vi "Register gRPC Messages.vi"(8 "error in (no error)":errorcluster, 11 "gRPC ID":T1) -> (0 "error out":errorcluster, 3 "gRPC ID Out":T1)   [LabVIEW 2021, in "NI_DAQmx_client.lvlib"]
uses:
  NI_DAQmx_client.lvlib
  <vilib>/gRPC/LabVIEW gRPC Library/Shared/grpcId.ctl
  <vilib>/gRPC/LabVIEW gRPC Library/Server API/typeDefs/Message Metadata.ctl
  <vilib>/gRPC/LabVIEW gRPC Library/Server API/typeDefs/Message Element Metadata.ctl
  <vilib>/gRPC/LabVIEW gRPC Library/Server API/typeDefs/Message Element Type.ctl
  <vilib>/gRPC/LabVIEW gRPC Library/Server API/typeDefs/Enum Metadata.ctl
  <vilib>/gRPC/LabVIEW gRPC Library/grpc-lvsupport-release.lvlib
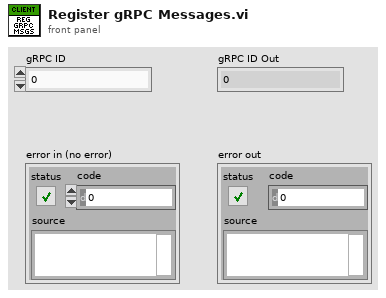
[diagram p1: front panel]
types:
  T1 = typedef "grpc-lvsupport-release.lvlib/grpcId.ctl" = u64
  T2 = typedef "grpc-lvsupport-release.lvlib/Enum Metadata.ctl" = cluster{"Version":i32, "Name":string, "Type Url":string, "Enum Values":string, "Allow Alias":bool}
  T3 = typedef "grpc-lvsupport-release.lvlib/Message Metadata.ctl" = cluster{"Version":i32, "Name":string, "Type Url":string, "Elements":T4[], "Has Oneof":bool}
  T4 = typedef "grpc-lvsupport-release.lvlib/Message Element Metadata.ctl" = cluster{"Field Name":string, "Embedded Message Name":string, "Protobuf Index":i32, "MessageElementType":T5, "Repeated":bool, "Is in Oneof":bool, "Oneof Container Name":string}
  T5 = typedef "grpc-lvsupport-release.lvlib/Message Element Type.ctl" = enum32{"Int32Value", "FloatValue", "DoubleValue", "BoolValue", "StringValue", "MessageValue", "Int64Value", "UInt32Value", "UInt64Value", "EnumValue", "Bytes", "Fixed64", "Fixed32", "SFixed64", "SFixed32", "SInt64", "SInt32"}
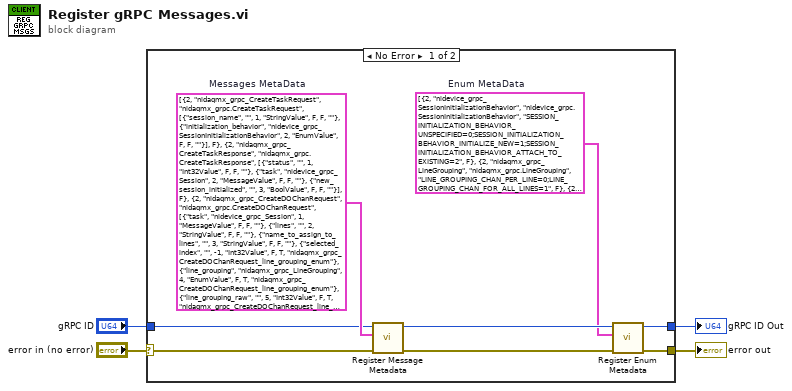
[diagram p0: block diagram]
diagram:
  n1 = case shown="No Error" "error in (no error)" {
    selector: "error in (no error)" -> [w10 w13]
    tunnel: [w9 w12] -> w1
    tunnel: [w6 w13] -> w4
    tunnel: "gRPC ID" -> [w9 w12]
    frame No Error {
      w5 = T2[] [{"Version"=2, "Name"="nidevice_grpc_SessionInitializationBehavior", "Type Url"="nidevice_grpc.SessionInitializationBehavior", "Enum Values"="SESSION_INITIALIZATION_BEHAVIOR_UNSPECIFIED=0;SESSION_INITIALIZATION_BEHAVIOR_INITIALIZE_NEW=1;SESSION_INITIALIZATION_BEHAVIOR_ATTACH_TO_EXISTING=2", "Allow Alias"=FALSE}, {"Version"=2, "Name"="nidaqmx_grpc_LineGrouping", "Type Url"="nidaqmx_grpc.LineGrouping", "Enum Values"="LINE_GROUPING_CHAN_PER_LINE=0;LINE_GROUPING_CHAN_FOR_ALL_LINES=1", "Allow Alias"=FALSE}, {"Version"=2, "Name"="nidaqmx_grpc_FrequencyUnits3", "Type Url"="nidaqmx_grpc.FrequencyUnits3", "Enum Values"="FREQUENCY_UNITS3_UNSPECIFIED=0;FREQUENCY_UNITS3_HZ=10373;FREQUENCY_UNITS3_TICKS=10304;FREQUENCY_UNITS3_FROM_CUSTOM_SCALE=10065", "Allow Alias"=FALSE}, {"Version"=2, "Name"="nidaqmx_grpc_Edge1", "Type Url"="nidaqmx_grpc.Edge1", "Enum Values"="EDGE1_UNSPECIFIED=0;EDGE1_RISING=10280;EDGE1_FALLING=10171", "Allow Alias"=FALSE}, {"Version"=2, "Name"="nidaqmx_grpc_CounterFrequencyMethod", "Type Url"="nidaqmx_grpc.CounterFrequencyMethod", "Enum Values"="COUNTER_FREQUENCY_METHOD_UNSPECIFIED=0;COUNTER_FREQUENCY_METHOD_LOW_FREQ_1_CTR=10105;COUNTER_FREQUENCY_METHOD_HIGH_FREQ_2_CTR=10157;COUNTER_FREQUENCY_METHOD_LARGE_RNG_2_CTR=10205;COUNTER_FREQUENCY_METHOD_DYN_AVG=16065", "Allow Alias"=FALSE}, {"Version"=2, "Name"="nidaqmx_grpc_GroupBy", "Type Url"="nidaqmx_grpc.GroupBy", "Enum Values"="GROUP_BY_GROUP_BY_CHANNEL=0;GROUP_BY_GROUP_BY_SCAN_NUMBER=1", "Allow Alias"=FALSE}, {"Version"=2, "Name"="nidaqmx_grpc_AcquisitionType", "Type Url"="nidaqmx_grpc.AcquisitionType", "Enum Values"="ACQUISITION_TYPE_UNSPECIFIED=0;ACQUISITION_TYPE_FINITE_SAMPS=10178;ACQUISITION_TYPE_CONT_SAMPS=10123;ACQUISITION_TYPE_HW_TIMED_SINGLE_POINT=12522", "Allow Alias"=FALSE}, {"Version"=2, "Name"="nidaqmx_grpc_TaskStringAttribute", "Type Url"="nidaqmx_grpc.TaskStringAttribute", "Enum Values"="TASK_STRING_ATTRIBUTE_UNSPECIFIED=0;TASK_ATTRIBUTE_CHANNELS=4723;TASK_ATTRIBUTE_NAME=4726;TASK_ATTRIBUTE_DEVICES=8974", "Allow Alias"=FALSE}, {"Version"=2, "Name"="nidaqmx_grpc_ChannelStringAttribute", "Type Url"="nidaqmx_grpc.ChannelStringAttribute", "Enum Values"="CHANNEL_STRING_ATTRIBUTE_UNSPECIFIED=0;CHANNEL_ATTRIBUTE_CI_CTR_TIMEBASE_SRC=323;CHANNEL_ATTRIBUTE_CO_CTR_TIMEBASE_SRC=825;CHANNEL_ATTRIBUTE_AI_THRMCPL_CJC_CHAN=4148;CHANNEL_ATTRIBUTE_CI_GPS_SYNC_SRC=4243;CHANNEL_ATTRIBUTE_AO_CUSTOM_SCALE_NAME=4488;CHANNEL_ATTRIBUTE_AI_CUSTOM_SCALE_NAME=6112;CHANNEL_ATTRIBUTE_CI_CUSTOM_SCALE_NAME=6302;CHANNEL_ATTRIBUTE_CI_FREQ_TERM=6306;CHANNEL_ATTRIBUTE_CI_PERIOD_TERM=6308;CHANNEL_ATTRIBUTE_CI_PULSE_WIDTH_TERM=6314;CHANNEL_ATTRIBUTE_CI_TWO_EDGE_SEP_FIRST_TERM=6317;CHANNEL_ATTRIBUTE_CI_TWO_EDGE_SEP_SECOND_TERM=6318;CHANNEL_ATTRIBUTE_CI_SEMI_PERIOD_TERM=6320;CHANNEL_ATTRIBUTE_CI_COUNT_EDGES_TERM=6343;CHANNEL_ATTRIBUTE_CO_PULSE_TERM=6369;CHANNEL_ATTRIBUTE_PHYSICAL_CHAN_NAME=6389;CHANNEL_ATTRIBUTE_CHAN_DESCR=6438;CHANNEL_ATTRIBUTE_AI_INPUT_SRC=8600;CHANNEL_ATTRIBUTE_CI_ENCODER_A_INPUT_TERM=8605;CHANNEL_ATTRIBUTE_CI_ENCODER_B_INPUT_TERM=8606;CHANNEL_ATTRIBUTE_CI_ENCODER_Z_INPUT_TERM=8607;CHANNEL_ATTRIBUTE_AI_TEDS_UNITS=8672;CHANNEL_ATTRIBUTE_CI_COUNT_EDGES_DIR_TERM=8673;CHANNEL_ATTRIBUTE_CI_FREQ_DIG_FLTR_TIMEBASE_SRC=8681;CHANNEL_ATTRIBUTE_CI_PERIOD_DIG_FLTR_TIMEBASE_SRC=8686;CHANNEL_ATTRIBUTE_CI_COUNT_EDGES_COUNT_DIR_DIG_FLTR_TIMEBASE_SRC=8691;CHANNEL_ATTRIBUTE_CI_COUNT_EDGES_DIG_FLTR_TIMEBASE_SRC=8696;CHANNEL_ATTRIBUTE_CI_ENCODER_A_INPUT_DIG_FLTR_TIMEBASE_SRC=8701;CHANNEL_ATTRIBUTE_CI_ENCODER_B_INPUT_DIG_FLTR_TIMEBASE_SRC=8706;CHANNEL_ATTRIBUTE_CI_ENCODER_Z_INPUT_DIG_FLTR_TIMEBASE_SRC=8711;CHANNEL_ATTRIBUTE_CI_PULSE_WIDTH_DIG_FLTR_TIMEBASE_SRC=8716;CHANNEL_ATTRIBUTE_CI_TWO_EDGE_SEP_FIRST_DIG_FLTR_TIMEBASE_SRC=8721;CHANNEL_ATTRIBUTE_CI_TWO_EDGE_SEP_SECOND_DIG_FLTR_TIMEBASE_SRC=8726;CHANNEL_ATTRIBUTE_CI_SEMI_PERIOD_DIG_FLTR_TIMEBASE_SRC=8731;CHANNEL_ATTRIBUTE_AO_DAC_REF_EXT_SRC=8786;CHANNEL_ATTRIBUTE_AO_DAC_OFFSET_EXT_SRC=8788;CHANNEL_ATTRIBUTE_CI_CTR_TIMEBASE_DIG_FLTR_TIMEBASE_SRC=8819;CHANNEL_ATTRIBUTE_CO_CTR_TIMEBASE_DIG_FLTR_TIMEBASE_SRC=8824;CHANNEL_ATTRIBUTE_AI_CHAN_CAL_OPERATOR_NAME=8867;CHANNEL_ATTRIBUTE_AI_CHAN_CAL_DESC=8868;CHANNEL_ATTRIBUTE_DI_DIG_FLTR_TIMEBASE_SRC=11988;CHANNEL_ATTRIBUTE_CI_PULSE_FREQ_TERM=12036;CHANNEL_ATTRIBUTE_CI_PULSE_FREQ_DIG_FLTR_TIMEBASE_SRC=12040;CHANNEL_ATTRIBUTE_CI_PULSE_TIME_TERM=12044;CHANNEL_ATTRIBUTE_CI_PULSE_TIME_DIG_FLTR_TIMEBASE_SRC=12048;CHANNEL_ATTRIBUTE_CI_PULSE_TICKS_TERM=12052;CHANNEL_ATTRIBUTE_CI_PULSE_TICKS_DIG_FLTR_TIMEBASE_SRC=12056;CHANNEL_ATTRIBUTE_CI_COUNT_EDGES_COUNT_RESET_TERM=12209;CHANNEL_ATTRIBUTE_CI_COUNT_EDGES_COUNT_RESET_DIG_FLTR_TIMEBASE_SRC=12213;CHANNEL_ATTRIBUTE_AI_ROSETTE_STRAIN_GAGE_STRAIN_CHANS=12283;CHANNEL_ATTRIBUTE_CI_TIMESTAMP_TERM=12345;CHANNEL_ATTRIBUTE_NAV_CUSTOM_SCALE_NAME=12348;CHANNEL_ATTRIBUTE_CI_DUTY_CYCLE_TERM=12429;CHANNEL_ATTRIBUTE_CI_DUTY_CYCLE_DIG_FLTR_TIMEBASE_SRC=12432;CHANNEL_ATTRIBUTE_CI_VELOCITY_ENCODER_A_INPUT_TERM=12509;CHANNEL_ATTRIBUTE_CI_VELOCITY_ENCODER_A_INPUT_DIG_FLTR_TIMEBASE_SRC=12514;CHANNEL_ATTRIBUTE_CI_VELOCITY_ENCODER_B_INPUT_TERM=12516;CHANNEL_ATTRIBUTE_CI_VELOCITY_ENCODER_B_INPUT_DIG_FLTR_TIMEBASE_SRC=12521;CHANNEL_ATTRIBUTE_CI_COUNT_EDGES_GATE_TERM=12526;CHANNEL_ATTRIBUTE_CI_COUNT_EDGES_GATE_DIG_FLTR_TIMEBASE_SRC=12531", "Allow Alias"=FALSE}, {"Version"=2, "Name"="nidaqmx_grpc_ChannelDoubleAttribute", "Type Url"="nidaqmx_grpc.ChannelDoubleAttribute", "Enum Values"="CHANNEL_DOUBLE_ATTRIBUTE_UNSPECIFIED=0;CHANNEL_ATTRIBUTE_AI_IMPEDANCE=98;CHANNEL_ATTRIBUTE_AI_AC_EXCIT_FREQ=257;CHANNEL_ATTRIBUTE_AO_GAIN=280;CHANNEL_ATTRIBUTE_AO_LOAD_IMPEDANCE=289;CHANNEL_ATTRIBUTE_CI_FREQ_MEAS_TIME=325;CHANNEL_ATTRIBUTE_CO_PULSE_FREQ_INITIAL_DELAY=665;CHANNEL_ATTRIBUTE_AI_ACCEL_SENSITIVITY=1682;CHANNEL_ATTRIBUTE_AI_FREQ_HYST=2068;CHANNEL_ATTRIBUTE_AI_FREQ_THRESH_VOLTAGE=2069;CHANNEL_ATTRIBUTE_CI_ANG_ENCODER_INITIAL_ANGLE=2177;CHANNEL_ATTRIBUTE_CI_ENCODER_Z_INDEX_VAL=2184;CHANNEL_ATTRIBUTE_AI_RVDT_SENSITIVITY=2307;CHANNEL_ATTRIBUTE_CI_LIN_ENCODER_DIST_PER_PULSE=2321;CHANNEL_ATTRIBUTE_CI_LIN_ENCODER_INITIAL_POS=2325;CHANNEL_ATTRIBUTE_AI_LVDT_SENSITIVITY=2361;CHANNEL_ATTRIBUTE_AI_STRAIN_GAGE_GAGE_FACTOR=2452;CHANNEL_ATTRIBUTE_AI_STRAIN_GAGE_POISSON_RATIO=2456;CHANNEL_ATTRIBUTE_AI_RTD_A=4112;CHANNEL_ATTRIBUTE_AI_RTD_B=4113;CHANNEL_ATTRIBUTE_AI_RTD_C=4115;CHANNEL_ATTRIBUTE_AI_RTD_R0=4144;CHANNEL_ATTRIBUTE_AI_THRMCPL_CJC_VAL=4150;CHANNEL_ATTRIBUTE_AI_THRMSTR_R1=4193;CHANNEL_ATTRIBUTE_CO_PULSE_DUTY_CYC=4470;CHANNEL_ATTRIBUTE_CO_PULSE_FREQ=4472;CHANNEL_ATTRIBUTE_AO_MAX=4486;CHANNEL_ATTRIBUTE_AO_MIN=4487;CHANNEL_ATTRIBUTE_AO_OUTPUT_IMPEDANCE=5264;CHANNEL_ATTRIBUTE_AI_MICROPHONE_SENSITIVITY=5430;CHANNEL_ATTRIBUTE_AI_RESOLUTION=5989;CHANNEL_ATTRIBUTE_AI_MAX=6109;CHANNEL_ATTRIBUTE_AI_MIN=6110;CHANNEL_ATTRIBUTE_AI_BRIDGE_NOM_RESISTANCE=6124;CHANNEL_ATTRIBUTE_AI_BRIDGE_INITIAL_VOLTAGE=6125;CHANNEL_ATTRIBUTE_AI_LEAD_WIRE_RESISTANCE=6126;CHANNEL_ATTRIBUTE_AI_CURRENT_SHUNT_RESISTANCE=6131;CHANNEL_ATTRIBUTE_AI_EXCIT_VAL=6133;CHANNEL_ATTRIBUTE_AI_ATTEN=6145;CHANNEL_ATTRIBUTE_AI_LOWPASS_CUTOFF_FREQ=6147;CHANNEL_ATTRIBUTE_AI_HIGHPASS_CUTOFF_FREQ=6151;CHANNEL_ATTRIBUTE_AI_BANDPASS_CENTER_FREQ=6156;CHANNEL_ATTRIBUTE_AI_BANDPASS_WIDTH=6158;CHANNEL_ATTRIBUTE_AI_NOTCH_CENTER_FREQ=6160;CHANNEL_ATTRIBUTE_AI_NOTCH_WIDTH=6162;CHANNEL_ATTRIBUTE_AI_RNG_HIGH=6165;CHANNEL_ATTRIBUTE_AI_RNG_LOW=6166;CHANNEL_ATTRIBUTE_AI_GAIN=6168;CHANNEL_ATTRIBUTE_AO_RESOLUTION=6188;CHANNEL_ATTRIBUTE_AO_DAC_RNG_LOW=6189;CHANNEL_ATTRIBUTE_AO_DAC_RNG_HIGH=6190;CHANNEL_ATTRIBUTE_AO_DAC_REF_VAL=6194;CHANNEL_ATTRIBUTE_AI_EXCIT_ACTUAL_VAL=6275;CHANNEL_ATTRIBUTE_AI_LOWPASS_SWITCH_CAP_EXT_CLK_FREQ=6277;CHANNEL_ATTRIBUTE_CI_MAX=6300;CHANNEL_ATTRIBUTE_CI_MIN=6301;CHANNEL_ATTRIBUTE_CI_CTR_TIMEBASE_RATE=6322;CHANNEL_ATTRIBUTE_CO_PULSE_HIGH_TIME=6330;CHANNEL_ATTRIBUTE_CO_PULSE_LOW_TIME=6331;CHANNEL_ATTRIBUTE_CO_PULSE_TIME_INITIAL_DELAY=6332;CHANNEL_ATTRIBUTE_CO_CTR_TIMEBASE_RATE=6338;CHANNEL_ATTRIBUTE_AI_THRMSTR_A=6345;CHANNEL_ATTRIBUTE_AI_THRMSTR_C=6346;CHANNEL_ATTRIBUTE_AI_THRMSTR_B=6347;CHANNEL_ATTRIBUTE_CI_PERIOD_MEAS_TIME=6445;CHANNEL_ATTRIBUTE_AI_BRIDGE_SHUNT_CAL_GAIN_ADJUST=6463;CHANNEL_ATTRIBUTE_DI_DIG_FLTR_MIN_PULSE_WIDTH=8663;CHANNEL_ATTRIBUTE_CI_FREQ_DIG_FLTR_MIN_PULSE_WIDTH=8680;CHANNEL_ATTRIBUTE_CI_FREQ_DIG_FLTR_TIMEBASE_RATE=8682;CHANNEL_ATTRIBUTE_CI_PERIOD_DIG_FLTR_MIN_PULSE_WIDTH=8685;CHANNEL_ATTRIBUTE_CI_PERIOD_DIG_FLTR_TIMEBASE_RATE=8687;CHANNEL_ATTRIBUTE_CI_COUNT_EDGES_COUNT_DIR_DIG_FLTR_MIN_PULSE_WIDTH=8690;CHANNEL_ATTRIBUTE_CI_COUNT_EDGES_COUNT_DIR_DIG_FLTR_TIMEBASE_RATE=8692;CHANNEL_ATTRIBUTE_CI_COUNT_EDGES_DIG_FLTR_MIN_PULSE_WIDTH=8695;CHANNEL_ATTRIBUTE_CI_COUNT_EDGES_DIG_FLTR_TIMEBASE_RATE=8697;CHANNEL_ATTRIBUTE_CI_ENCODER_A_INPUT_DIG_FLTR_MIN_PULSE_WIDTH=8700;CHANNEL_ATTRIBUTE_CI_ENCODER_A_INPUT_DIG_FLTR_TIMEBASE_RATE=8702;CHANNEL_ATTRIBUTE_CI_ENCODER_B_INPUT_DIG_FLTR_MIN_PULSE_WIDTH=8705;CHANNEL_ATTRIBUTE_CI_ENCODER_B_INPUT_DIG_FLTR_TIMEBASE_RATE=8707;CHANNEL_ATTRIBUTE_CI_ENCODER_Z_INPUT_DIG_FLTR_MIN_PULSE_WIDTH=8710;CHANNEL_ATTRIBUTE_CI_ENCODER_Z_INPUT_DIG_FLTR_TIMEBASE_RATE=8712;CHANNEL_ATTRIBUTE_CI_PULSE_WIDTH_DIG_FLTR_MIN_PULSE_WIDTH=8715;CHANNEL_ATTRIBUTE_CI_PULSE_WIDTH_DIG_FLTR_TIMEBASE_RATE=8717;CHANNEL_ATTRIBUTE_CI_TWO_EDGE_SEP_FIRST_DIG_FLTR_MIN_PULSE_WIDTH=8720;CHANNEL_ATTRIBUTE_CI_TWO_EDGE_SEP_FIRST_DIG_FLTR_TIMEBASE_RATE=8722;CHANNEL_ATTRIBUTE_CI_TWO_EDGE_SEP_SECOND_DIG_FLTR_MIN_PULSE_WIDTH=8725;CHANNEL_ATTRIBUTE_CI_TWO_EDGE_SEP_SECOND_DIG_FLTR_TIMEBASE_RATE=8727;CHANNEL_ATTRIBUTE_CI_SEMI_PERIOD_DIG_FLTR_MIN_PULSE_WIDTH=8730;CHANNEL_ATTRIBUTE_CI_SEMI_PERIOD_DIG_FLTR_TIMEBASE_RATE=8732;CHANNEL_ATTRIBUTE_AI_SOUND_PRESSURE_MAX_SOUND_PRESSURE_LVL=8762;CHANNEL_ATTRIBUTE_AO_DAC_OFFSET_VAL=8789;CHANNEL_ATTRIBUTE_CI_CTR_TIMEBASE_DIG_FLTR_MIN_PULSE_WIDTH=8818;CHANNEL_ATTRIBUTE_CI_CTR_TIMEBASE_DIG_FLTR_TIMEBASE_RATE=8820;CHANNEL_ATTRIBUTE_CO_CTR_TIMEBASE_DIG_FLTR_MIN_PULSE_WIDTH=8823;CHANNEL_ATTRIBUTE_CO_CTR_TIMEBASE_DIG_FLTR_TIMEBASE_RATE=8825;CHANNEL_ATTRIBUTE_AI_VOLTAGE_DB_REF=10672;CHANNEL_ATTRIBUTE_AI_SOUND_PRESSURE_DB_REF=10673;CHANNEL_ATTRIBUTE_AI_ACCEL_DB_REF=10674;CHANNEL_ATTRIBUTE_AO_FUNC_GEN_FREQ=10777;CHANNEL_ATTRIBUTE_AO_FUNC_GEN_AMPLITUDE=10778;CHANNEL_ATTRIBUTE_AO_FUNC_GEN_OFFSET=10779;CHANNEL_ATTRIBUTE_AO_FUNC_GEN_SQUARE_DUTY_CYCLE=10780;CHANNEL_ATTRIBUTE_AO_VOLTAGE_CURRENT_LIMIT=10781;CHANNEL_ATTRIBUTE_AO_FUNC_GEN_FM_DEVIATION=10787;CHANNEL_ATTRIBUTE_DO_OVERCURRENT_LIMIT=10885;CHANNEL_ATTRIBUTE_DO_OVERCURRENT_REENABLE_PERIOD=10887;CHANNEL_ATTRIBUTE_AI_PROBE_ATTEN=10888;CHANNEL_ATTRIBUTE_AI_DC_OFFSET=10889;CHANNEL_ATTRIBUTE_AI_EDDY_CURRENT_PROX_PROBE_SENSITIVITY=10942;CHANNEL_ATTRIBUTE_DI_DIG_FLTR_TIMEBASE_RATE=11989;CHANNEL_ATTRIBUTE_CI_PULSE_FREQ_DIG_FLTR_MIN_PULSE_WIDTH=12039;CHANNEL_ATTRIBUTE_CI_PULSE_FREQ_DIG_FLTR_TIMEBASE_RATE=12041;CHANNEL_ATTRIBUTE_CI_PULSE_TIME_DIG_FLTR_MIN_PULSE_WIDTH=12047;CHANNEL_ATTRIBUTE_CI_PULSE_TIME_DIG_FLTR_TIMEBASE_RATE=12049;CHANNEL_ATTRIBUTE_CI_PULSE_TICKS_DIG_FLTR_MIN_PULSE_WIDTH=12055;CHANNEL_ATTRIBUTE_CI_PULSE_TICKS_DIG_FLTR_TIMEBASE_RATE=12057;CHANNEL_ATTRIBUTE_AI_BRIDGE_SHUNT_CAL_SHUNT_CAL_A_RESISTANCE=12152;CHANNEL_ATTRIBUTE_AI_BRIDGE_SHUNT_CAL_SHUNT_CAL_A_ACTUAL_RESISTANCE=12153;CHANNEL_ATTRIBUTE_AI_BRIDGE_SHUNT_CAL_SHUNT_CAL_B_RESISTANCE=12154;CHANNEL_ATTRIBUTE_AI_BRIDGE_SHUNT_CAL_SHUNT_CAL_B_ACTUAL_RESISTANCE=12155;CHANNEL_ATTRIBUTE_AI_FORCE_IEPE_SENSOR_SENSITIVITY=12161;CHANNEL_ATTRIBUTE_AI_BRIDGE_INITIAL_RATIO=12166;CHANNEL_ATTRIBUTE_AI_BRIDGE_TWO_POINT_LIN_FIRST_ELECTRICAL_VAL=12170;CHANNEL_ATTRIBUTE_AI_BRIDGE_TWO_POINT_LIN_FIRST_PHYSICAL_VAL=12171;CHANNEL_ATTRIBUTE_AI_BRIDGE_TWO_POINT_LIN_SECOND_ELECTRICAL_VAL=12172;CHANNEL_ATTRIBUTE_AI_BRIDGE_TWO_POINT_LIN_SECOND_PHYSICAL_VAL=12173;CHANNEL_ATTRIBUTE_CI_COUNT_EDGES_COUNT_RESET_DIG_FLTR_MIN_PULSE_WIDTH=12212;CHANNEL_ATTRIBUTE_CI_COUNT_EDGES_COUNT_RESET_DIG_FLTR_TIMEBASE_RATE=12214;CHANNEL_ATTRIBUTE_AI_THRMCPL_LEAD_OFFSET_VOLTAGE=12216;CHANNEL_ATTRIBUTE_AI_FILTER_DELAY=12269;CHANNEL_ATTRIBUTE_AI_VELOCITY_IEPE_SENSOR_DB_REF=12277;CHANNEL_ATTRIBUTE_AI_VELOCITY_IEPE_SENSOR_SENSITIVITY=12278;CHANNEL_ATTRIBUTE_AI_ROSETTE_STRAIN_GAGE_ORIENTATION=12284;CHANNEL_ATTRIBUTE_AO_FILTER_DELAY_ADJUSTMENT=12402;CHANNEL_ATTRIBUTE_AI_FILTER_DELAY_ADJUSTMENT=12404;CHANNEL_ATTRIBUTE_AO_FILTER_DELAY=12405;CHANNEL_ATTRIBUTE_CI_DUTY_CYCLE_DIG_FLTR_MIN_PULSE_WIDTH=12431;CHANNEL_ATTRIBUTE_CI_DUTY_CYCLE_DIG_FLTR_TIMEBASE_RATE=12433;CHANNEL_ATTRIBUTE_CI_MAX_MEAS_PERIOD=12437;CHANNEL_ATTRIBUTE_CI_THRESH_VOLTAGE=12471;CHANNEL_ATTRIBUTE_AI_DIG_FLTR_LOWPASS_CUTOFF_FREQ=12481;CHANNEL_ATTRIBUTE_AI_DIG_FLTR_HIGHPASS_CUTOFF_FREQ=12482;CHANNEL_ATTRIBUTE_AI_DIG_FLTR_BANDPASS_CENTER_FREQ=12483;CHANNEL_ATTRIBUTE_AI_DIG_FLTR_BANDPASS_WIDTH=12484;CHANNEL_ATTRIBUTE_AI_DIG_FLTR_NOTCH_CENTER_FREQ=12485;CHANNEL_ATTRIBUTE_AI_DIG_FLTR_NOTCH_WIDTH=12486;CHANNEL_ATTRIBUTE_CI_VELOCITY_LIN_ENCODER_DIST_PER_PULSE=12507;CHANNEL_ATTRIBUTE_CI_VELOCITY_ENCODER_A_INPUT_DIG_FLTR_MIN_PULSE_WIDTH=12513;CHANNEL_ATTRIBUTE_CI_VELOCITY_ENCODER_A_INPUT_DIG_FLTR_TIMEBASE_RATE=12515;CHANNEL_ATTRIBUTE_CI_VELOCITY_ENCODER_B_INPUT_DIG_FLTR_MIN_PULSE_WIDTH=12520;CHANNEL_ATTRIBUTE_CI_VELOCITY_ENCODER_B_INPUT_DIG_FLTR_TIMEBASE_RATE=12522;CHANNEL_ATTRIBUTE_CI_VELOCITY_MEAS_TIME=12523;CHANNEL_ATTRIBUTE_CI_COUNT_EDGES_GATE_DIG_FLTR_MIN_PULSE_WIDTH=12530;CHANNEL_ATTRIBUTE_CI_COUNT_EDGES_GATE_DIG_FLTR_TIMEBASE_RATE=12532;CHANNEL_ATTRIBUTE_AI_ACCEL_CHARGE_SENSITIVITY=12563;CHANNEL_ATTRIBUTE_AI_ACCEL_4_WIRE_DC_VOLTAGE_SENSITIVITY=12565;CHANNEL_ATTRIBUTE_AI_DATA_XFER_MAX_RATE=12567;CHANNEL_ATTRIBUTE_AI_SENSOR_POWER_VOLTAGE=12649;CHANNEL_ATTRIBUTE_AI_FILTER_FREQ=12660;CHANNEL_ATTRIBUTE_AI_INPUT_LIMITS_FAULT_DETECT_UPPER_LIMIT=12684;CHANNEL_ATTRIBUTE_AI_INPUT_LIMITS_FAULT_DETECT_LOWER_LIMIT=12685;CHANNEL_ATTRIBUTE_CI_FREQ_THRESH_VOLTAGE=12715;CHANNEL_ATTRIBUTE_CI_FREQ_HYST=12716;CHANNEL_ATTRIBUTE_CI_PERIOD_THRESH_VOLTAGE=12717;CHANNEL_ATTRIBUTE_CI_PERIOD_HYST=12718;CHANNEL_ATTRIBUTE_CI_COUNT_EDGES_THRESH_VOLTAGE=12719;CHANNEL_ATTRIBUTE_CI_COUNT_EDGES_HYST=12720;CHANNEL_ATTRIBUTE_CI_COUNT_EDGES_COUNT_DIR_THRESH_VOLTAGE=12721;CHANNEL_ATTRIBUTE_CI_COUNT_EDGES_COUNT_DIR_HYST=12722;CHANNEL_ATTRIBUTE_CI_COUNT_EDGES_COUNT_RESET_THRESH_VOLTAGE=12723;CHANNEL_ATTRIBUTE_CI_COUNT_EDGES_COUNT_RESET_HYST=12724;CHANNEL_ATTRIBUTE_CI_COUNT_EDGES_GATE_THRESH_VOLTAGE=12725;CHANNEL_ATTRIBUTE_CI_COUNT_EDGES_GATE_HYST=12726;CHANNEL_ATTRIBUTE_CI_FILTER_FREQ=12728;CHANNEL_ATTRIBUTE_CI_FILTER_DELAY=12731;CHANNEL_ATTRIBUTE_AO_FUNC_GEN_START_PHASE=12740;CHANNEL_ATTRIBUTE_AO_COMMON_MODE_OFFSET=12748;CHANNEL_ATTRIBUTE_PWR_VOLTAGE_SETPOINT=12756;CHANNEL_ATTRIBUTE_PWR_CURRENT_SETPOINT=12757", "Allow Alias"=FALSE}]  # Enum MetaData
      w11 = T3[] [{"Version"=2, "Name"="nidaqmx_grpc_CreateTaskRequest", "Type Url"="nidaqmx_grpc.CreateTaskRequest", "Elements"=[{"Field Name"="session_name", "Embedded Message Name"="", "Protobuf Index"=1, "MessageElementType"=enum."StringValue", "Repeated"=FALSE, "Is in Oneof"=FALSE, "Oneof Container Name"=""}, {"Field Name"="initialization_behavior", "Embedded Message Name"="nidevice_grpc_SessionInitializationBehavior", "Protobuf Index"=2, "MessageElementType"=enum."EnumValue", "Repeated"=FALSE, "Is in Oneof"=FALSE, "Oneof Container Name"=""}], "Has Oneof"=FALSE}, {"Version"=2, "Name"="nidaqmx_grpc_CreateTaskResponse", "Type Url"="nidaqmx_grpc.CreateTaskResponse", "Elements"=[{"Field Name"="status", "Embedded Message Name"="", "Protobuf Index"=1, "MessageElementType"=enum."Int32Value", "Repeated"=FALSE, "Is in Oneof"=FALSE, "Oneof Container Name"=""}, {"Field Name"="task", "Embedded Message Name"="nidevice_grpc_Session", "Protobuf Index"=2, "MessageElementType"=enum."MessageValue", "Repeated"=FALSE, "Is in Oneof"=FALSE, "Oneof Container Name"=""}, {"Field Name"="new_session_initialized", "Embedded Message Name"="", "Protobuf Index"=3, "MessageElementType"=enum."BoolValue", "Repeated"=FALSE, "Is in Oneof"=FALSE, "Oneof Container Name"=""}], "Has Oneof"=FALSE}, {"Version"=2, "Name"="nidaqmx_grpc_CreateDOChanRequest", "Type Url"="nidaqmx_grpc.CreateDOChanRequest", "Elements"=[{"Field Name"="task", "Embedded Message Name"="nidevice_grpc_Session", "Protobuf Index"=1, "MessageElementType"=enum."MessageValue", "Repeated"=FALSE, "Is in Oneof"=FALSE, "Oneof Container Name"=""}, {"Field Name"="lines", "Embedded Message Name"="", "Protobuf Index"=2, "MessageElementType"=enum."StringValue", "Repeated"=FALSE, "Is in Oneof"=FALSE, "Oneof Container Name"=""}, {"Field Name"="name_to_assign_to_lines", "Embedded Message Name"="", "Protobuf Index"=3, "MessageElementType"=enum."StringValue", "Repeated"=FALSE, "Is in Oneof"=FALSE, "Oneof Container Name"=""}, {"Field Name"="selected_index", "Embedded Message Name"="", "Protobuf Index"=-1, "MessageElementType"=enum."Int32Value", "Repeated"=FALSE, "Is in Oneof"=TRUE, "Oneof Container Name"="nidaqmx_grpc_CreateDOChanRequest_line_grouping_enum"}, {"Field Name"="line_grouping", "Embedded Message Name"="nidaqmx_grpc_LineGrouping", "Protobuf Index"=4, "MessageElementType"=enum."EnumValue", "Repeated"=FALSE, "Is in Oneof"=TRUE, "Oneof Container Name"="nidaqmx_grpc_CreateDOChanRequest_line_grouping_enum"}, {"Field Name"="line_grouping_raw", "Embedded Message Name"="", "Protobuf Index"=5, "MessageElementType"=enum."Int32Value", "Repeated"=FALSE, "Is in Oneof"=TRUE, "Oneof Container Name"="nidaqmx_grpc_CreateDOChanRequest_line_grouping_enum"}], "Has Oneof"=TRUE}, {"Version"=2, "Name"="nidaqmx_grpc_CreateDOChanResponse", "Type Url"="nidaqmx_grpc.CreateDOChanResponse", "Elements"=[{"Field Name"="status", "Embedded Message Name"="", "Protobuf Index"=1, "MessageElementType"=enum."Int32Value", "Repeated"=FALSE, "Is in Oneof"=FALSE, "Oneof Container Name"=""}], "Has Oneof"=FALSE}, {"Version"=2, "Name"="nidaqmx_grpc_CreateCIFreqChanRequest", "Type Url"="nidaqmx_grpc.CreateCIFreqChanRequest", "Elements"=[{"Field Name"="task", "Embedded Message Name"="nidevice_grpc_Session", "Protobuf Index"=1, "MessageElementType"=enum."MessageValue", "Repeated"=FALSE, "Is in Oneof"=FALSE, "Oneof Container Name"=""}, {"Field Name"="counter", "Embedded Message Name"="", "Protobuf Index"=2, "MessageElementType"=enum."StringValue", "Repeated"=FALSE, "Is in Oneof"=FALSE, "Oneof Container Name"=""}, {"Field Name"="name_to_assign_to_channel", "Embedded Message Name"="", "Protobuf Index"=3, "MessageElementType"=enum."StringValue", "Repeated"=FALSE, "Is in Oneof"=FALSE, "Oneof Container Name"=""}, {"Field Name"="min_val", "Embedded Message Name"="", "Protobuf Index"=4, "MessageElementType"=enum."DoubleValue", "Repeated"=FALSE, "Is in Oneof"=FALSE, "Oneof Container Name"=""}, {"Field Name"="max_val", "Embedded Message Name"="", "Protobuf Index"=5, "MessageElementType"=enum."DoubleValue", "Repeated"=FALSE, "Is in Oneof"=FALSE, "Oneof Container Name"=""}, {"Field Name"="selected_index", "Embedded Message Name"="", "Protobuf Index"=-1, "MessageElementType"=enum."Int32Value", "Repeated"=FALSE, "Is in Oneof"=TRUE, "Oneof Container Name"="nidaqmx_grpc_CreateCIFreqChanRequest_units_enum"}, {"Field Name"="units", "Embedded Message Name"="nidaqmx_grpc_FrequencyUnits3", "Protobuf Index"=6, "MessageElementType"=enum."EnumValue", "Repeated"=FALSE, "Is in Oneof"=TRUE, "Oneof Container Name"="nidaqmx_grpc_CreateCIFreqChanRequest_units_enum"}, {"Field Name"="units_raw", "Embedded Message Name"="", "Protobuf Index"=7, "MessageElementType"=enum."Int32Value", "Repeated"=FALSE, "Is in Oneof"=TRUE, "Oneof Container Name"="nidaqmx_grpc_CreateCIFreqChanRequest_units_enum"}, {"Field Name"="selected_index", "Embedded Message Name"="", "Protobuf Index"=-1, "MessageElementType"=enum."Int32Value", "Repeated"=FALSE, "Is in Oneof"=TRUE, "Oneof Container Name"="nidaqmx_grpc_CreateCIFreqChanRequest_edge_enum"}, {"Field Name"="edge", "Embedded Message Name"="nidaqmx_grpc_Edge1", "Protobuf Index"=8, "MessageElementType"=enum."EnumValue", "Repeated"=FALSE, "Is in Oneof"=TRUE, "Oneof Container Name"="nidaqmx_grpc_CreateCIFreqChanRequest_edge_enum"}, {"Field Name"="edge_raw", "Embedded Message Name"="", "Protobuf Index"=9, "MessageElementType"=enum."Int32Value", "Repeated"=FALSE, "Is in Oneof"=TRUE, "Oneof Container Name"="nidaqmx_grpc_CreateCIFreqChanRequest_edge_enum"}, {"Field Name"="selected_index", "Embedded Message Name"="", "Protobuf Index"=-1, "MessageElementType"=enum."Int32Value", "Repeated"=FALSE, "Is in Oneof"=TRUE, "Oneof Container Name"="nidaqmx_grpc_CreateCIFreqChanRequest_meas_method_enum"}, {"Field Name"="meas_method", "Embedded Message Name"="nidaqmx_grpc_CounterFrequencyMethod", "Protobuf Index"=10, "MessageElementType"=enum."EnumValue", "Repeated"=FALSE, "Is in Oneof"=TRUE, "Oneof Container Name"="nidaqmx_grpc_CreateCIFreqChanRequest_meas_method_enum"}, {"Field Name"="meas_method_raw", "Embedded Message Name"="", "Protobuf Index"=11, "MessageElementType"=enum."Int32Value", "Repeated"=FALSE, "Is in Oneof"=TRUE, "Oneof Container Name"="nidaqmx_grpc_CreateCIFreqChanRequest_meas_method_enum"}, {"Field Name"="meas_time", "Embedded Message Name"="", "Protobuf Index"=12, "MessageElementType"=enum."DoubleValue", "Repeated"=FALSE, "Is in Oneof"=FALSE, "Oneof Container Name"=""}, {"Field Name"="divisor", "Embedded Message Name"="", "Protobuf Index"=13, "MessageElementType"=enum."UInt32Value", "Repeated"=FALSE, "Is in Oneof"=FALSE, "Oneof Container Name"=""}, {"Field Name"="custom_scale_name", "Embedded Message Name"="", "Protobuf Index"=14, "MessageElementType"=enum."StringValue", "Repeated"=FALSE, "Is in Oneof"=FALSE, "Oneof Container Name"=""}], "Has Oneof"=TRUE}, {"Version"=2, "Name"="nidaqmx_grpc_CreateCIFreqChanResponse", "Type Url"="nidaqmx_grpc.CreateCIFreqChanResponse", "Elements"=[{"Field Name"="status", "Embedded Message Name"="", "Protobuf Index"=1, "MessageElementType"=enum."Int32Value", "Repeated"=FALSE, "Is in Oneof"=FALSE, "Oneof Container Name"=""}], "Has Oneof"=FALSE}, {"Version"=2, "Name"="nidaqmx_grpc_WriteDigitalLinesRequest", "Type Url"="nidaqmx_grpc.WriteDigitalLinesRequest", "Elements"=[{"Field Name"="task", "Embedded Message Name"="nidevice_grpc_Session", "Protobuf Index"=1, "MessageElementType"=enum."MessageValue", "Repeated"=FALSE, "Is in Oneof"=FALSE, "Oneof Container Name"=""}, {"Field Name"="num_samps_per_chan", "Embedded Message Name"="", "Protobuf Index"=2, "MessageElementType"=enum."Int32Value", "Repeated"=FALSE, "Is in Oneof"=FALSE, "Oneof Container Name"=""}, {"Field Name"="auto_start", "Embedded Message Name"="", "Protobuf Index"=3, "MessageElementType"=enum."BoolValue", "Repeated"=FALSE, "Is in Oneof"=FALSE, "Oneof Container Name"=""}, {"Field Name"="timeout", "Embedded Message Name"="", "Protobuf Index"=4, "MessageElementType"=enum."DoubleValue", "Repeated"=FALSE, "Is in Oneof"=FALSE, "Oneof Container Name"=""}, {"Field Name"="selected_index", "Embedded Message Name"="", "Protobuf Index"=-1, "MessageElementType"=enum."Int32Value", "Repeated"=FALSE, "Is in Oneof"=TRUE, "Oneof Container Name"="nidaqmx_grpc_WriteDigitalLinesRequest_data_layout_enum"}, {"Field Name"="data_layout", "Embedded Message Name"="nidaqmx_grpc_GroupBy", "Protobuf Index"=5, "MessageElementType"=enum."EnumValue", "Repeated"=FALSE, "Is in Oneof"=TRUE, "Oneof Container Name"="nidaqmx_grpc_WriteDigitalLinesRequest_data_layout_enum"}, {"Field Name"="data_layout_raw", "Embedded Message Name"="", "Protobuf Index"=6, "MessageElementType"=enum."Int32Value", "Repeated"=FALSE, "Is in Oneof"=TRUE, "Oneof Container Name"="nidaqmx_grpc_WriteDigitalLinesRequest_data_layout_enum"}, {"Field Name"="write_array", "Embedded Message Name"="", "Protobuf Index"=7, "MessageElementType"=enum."Bytes", "Repeated"=FALSE, "Is in Oneof"=FALSE, "Oneof Container Name"=""}], "Has Oneof"=TRUE}, {"Version"=2, "Name"="nidaqmx_grpc_WriteDigitalLinesResponse", "Type Url"="nidaqmx_grpc.WriteDigitalLinesResponse", "Elements"=[{"Field Name"="status", "Embedded Message Name"="", "Protobuf Index"=1, "MessageElementType"=enum."Int32Value", "Repeated"=FALSE, "Is in Oneof"=FALSE, "Oneof Container Name"=""}, {"Field Name"="samps_per_chan_written", "Embedded Message Name"="", "Protobuf Index"=2, "MessageElementType"=enum."Int32Value", "Repeated"=FALSE, "Is in Oneof"=FALSE, "Oneof Container Name"=""}], "Has Oneof"=FALSE}, {"Version"=2, "Name"="nidaqmx_grpc_ReadCounterScalarF64Request", "Type Url"="nidaqmx_grpc.ReadCounterScalarF64Request", "Elements"=[{"Field Name"="task", "Embedded Message Name"="nidevice_grpc_Session", "Protobuf Index"=1, "MessageElementType"=enum."MessageValue", "Repeated"=FALSE, "Is in Oneof"=FALSE, "Oneof Container Name"=""}, {"Field Name"="timeout", "Embedded Message Name"="", "Protobuf Index"=2, "MessageElementType"=enum."DoubleValue", "Repeated"=FALSE, "Is in Oneof"=FALSE, "Oneof Container Name"=""}], "Has Oneof"=FALSE}, {"Version"=2, "Name"="nidaqmx_grpc_ReadCounterScalarF64Response", "Type Url"="nidaqmx_grpc.ReadCounterScalarF64Response", "Elements"=[{"Field Name"="status", "Embedded Message Name"="", "Protobuf Index"=1, "MessageElementType"=enum."Int32Value", "Repeated"=FALSE, "Is in Oneof"=FALSE, "Oneof Container Name"=""}, {"Field Name"="value", "Embedded Message Name"="", "Protobuf Index"=2, "MessageElementType"=enum."DoubleValue", "Repeated"=FALSE, "Is in Oneof"=FALSE, "Oneof Container Name"=""}], "Has Oneof"=FALSE}, {"Version"=2, "Name"="nidaqmx_grpc_CfgImplicitTimingRequest", "Type Url"="nidaqmx_grpc.CfgImplicitTimingRequest", "Elements"=[{"Field Name"="task", "Embedded Message Name"="nidevice_grpc_Session", "Protobuf Index"=1, "MessageElementType"=enum."MessageValue", "Repeated"=FALSE, "Is in Oneof"=FALSE, "Oneof Container Name"=""}, {"Field Name"="selected_index", "Embedded Message Name"="", "Protobuf Index"=-1, "MessageElementType"=enum."Int32Value", "Repeated"=FALSE, "Is in Oneof"=TRUE, "Oneof Container Name"="nidaqmx_grpc_CfgImplicitTimingRequest_sample_mode_enum"}, {"Field Name"="sample_mode", "Embedded Message Name"="nidaqmx_grpc_AcquisitionType", "Protobuf Index"=2, "MessageElementType"=enum."EnumValue", "Repeated"=FALSE, "Is in Oneof"=TRUE, "Oneof Container Name"="nidaqmx_grpc_CfgImplicitTimingRequest_sample_mode_enum"}, {"Field Name"="sample_mode_raw", "Embedded Message Name"="", "Protobuf Index"=3, "MessageElementType"=enum."Int32Value", "Repeated"=FALSE, "Is in Oneof"=TRUE, "Oneof Container Name"="nidaqmx_grpc_CfgImplicitTimingRequest_sample_mode_enum"}, {"Field Name"="samps_per_chan", "Embedded Message Name"="", "Protobuf Index"=4, "MessageElementType"=enum."UInt64Value", "Repeated"=FALSE, "Is in Oneof"=FALSE, "Oneof Container Name"=""}], "Has Oneof"=TRUE}, {"Version"=2, "Name"="nidaqmx_grpc_CfgImplicitTimingResponse", "Type Url"="nidaqmx_grpc.CfgImplicitTimingResponse", "Elements"=[{"Field Name"="status", "Embedded Message Name"="", "Protobuf Index"=1, "MessageElementType"=enum."Int32Value", "Repeated"=FALSE, "Is in Oneof"=FALSE, "Oneof Container Name"=""}], "Has Oneof"=FALSE}, {"Version"=2, "Name"="nidaqmx_grpc_StartTaskRequest", "Type Url"="nidaqmx_grpc.StartTaskRequest", "Elements"=[{"Field Name"="task", "Embedded Message Name"="nidevice_grpc_Session", "Protobuf Index"=1, "MessageElementType"=enum."MessageValue", "Repeated"=FALSE, "Is in Oneof"=FALSE, "Oneof Container Name"=""}], "Has Oneof"=FALSE}, {"Version"=2, "Name"="nidaqmx_grpc_StartTaskResponse", "Type Url"="nidaqmx_grpc.StartTaskResponse", "Elements"=[{"Field Name"="status", "Embedded Message Name"="", "Protobuf Index"=1, "MessageElementType"=enum."Int32Value", "Repeated"=FALSE, "Is in Oneof"=FALSE, "Oneof Container Name"=""}], "Has Oneof"=FALSE}, {"Version"=2, "Name"="nidaqmx_grpc_StopTaskRequest", "Type Url"="nidaqmx_grpc.StopTaskRequest", "Elements"=[{"Field Name"="task", "Embedded Message Name"="nidevice_grpc_Session", "Protobuf Index"=1, "MessageElementType"=enum."MessageValue", "Repeated"=FALSE, "Is in Oneof"=FALSE, "Oneof Container Name"=""}], "Has Oneof"=FALSE}, {"Version"=2, "Name"="nidaqmx_grpc_StopTaskResponse", "Type Url"="nidaqmx_grpc.StopTaskResponse", "Elements"=[{"Field Name"="status", "Embedded Message Name"="", "Protobuf Index"=1, "MessageElementType"=enum."Int32Value", "Repeated"=FALSE, "Is in Oneof"=FALSE, "Oneof Container Name"=""}], "Has Oneof"=FALSE}, {"Version"=2, "Name"="nidaqmx_grpc_ClearTaskRequest", "Type Url"="nidaqmx_grpc.ClearTaskRequest", "Elements"=[{"Field Name"="task", "Embedded Message Name"="nidevice_grpc_Session", "Protobuf Index"=1, "MessageElementType"=enum."MessageValue", "Repeated"=FALSE, "Is in Oneof"=FALSE, "Oneof Container Name"=""}], "Has Oneof"=FALSE}, {"Version"=2, "Name"="nidaqmx_grpc_ClearTaskResponse", "Type Url"="nidaqmx_grpc.ClearTaskResponse", "Elements"=[{"Field Name"="status", "Embedded Message Name"="", "Protobuf Index"=1, "MessageElementType"=enum."Int32Value", "Repeated"=FALSE, "Is in Oneof"=FALSE, "Oneof Container Name"=""}], "Has Oneof"=FALSE}, {"Version"=2, "Name"="nidaqmx_grpc_GetTaskAttributeStringRequest", "Type Url"="nidaqmx_grpc.GetTaskAttributeStringRequest", "Elements"=[{"Field Name"="task", "Embedded Message Name"="nidevice_grpc_Session", "Protobuf Index"=1, "MessageElementType"=enum."MessageValue", "Repeated"=FALSE, "Is in Oneof"=FALSE, "Oneof Container Name"=""}, {"Field Name"="selected_index", "Embedded Message Name"="", "Protobuf Index"=-1, "MessageElementType"=enum."Int32Value", "Repeated"=FALSE, "Is in Oneof"=TRUE, "Oneof Container Name"="nidaqmx_grpc_GetTaskAttributeStringRequest_attribute_enum"}, {"Field Name"="attribute", "Embedded Message Name"="nidaqmx_grpc_TaskStringAttribute", "Protobuf Index"=2, "MessageElementType"=enum."EnumValue", "Repeated"=FALSE, "Is in Oneof"=TRUE, "Oneof Container Name"="nidaqmx_grpc_GetTaskAttributeStringRequest_attribute_enum"}, {"Field Name"="attribute_raw", "Embedded Message Name"="", "Protobuf Index"=3, "MessageElementType"=enum."Int32Value", "Repeated"=FALSE, "Is in Oneof"=TRUE, "Oneof Container Name"="nidaqmx_grpc_GetTaskAttributeStringRequest_attribute_enum"}], "Has Oneof"=TRUE}, {"Version"=2, "Name"="nidaqmx_grpc_GetTaskAttributeStringResponse", "Type Url"="nidaqmx_grpc.GetTaskAttributeStringResponse", "Elements"=[{"Field Name"="status", "Embedded Message Name"="", "Protobuf Index"=1, "MessageElementType"=enum."Int32Value", "Repeated"=FALSE, "Is in Oneof"=FALSE, "Oneof Container Name"=""}, {"Field Name"="value", "Embedded Message Name"="", "Protobuf Index"=2, "MessageElementType"=enum."StringValue", "Repeated"=FALSE, "Is in Oneof"=FALSE, "Oneof Container Name"=""}], "Has Oneof"=FALSE}, {"Version"=2, "Name"="nidaqmx_grpc_GetChanAttributeStringRequest", "Type Url"="nidaqmx_grpc.GetChanAttributeStringRequest", "Elements"=[{"Field Name"="task", "Embedded Message Name"="nidevice_grpc_Session", "Protobuf Index"=1, "MessageElementType"=enum."MessageValue", "Repeated"=FALSE, "Is in Oneof"=FALSE, "Oneof Container Name"=""}, {"Field Name"="channel", "Embedded Message Name"="", "Protobuf Index"=2, "MessageElementType"=enum."StringValue", "Repeated"=FALSE, "Is in Oneof"=FALSE, "Oneof Container Name"=""}, {"Field Name"="selected_index", "Embedded Message Name"="", "Protobuf Index"=-1, "MessageElementType"=enum."Int32Value", "Repeated"=FALSE, "Is in Oneof"=TRUE, "Oneof Container Name"="nidaqmx_grpc_GetChanAttributeStringRequest_attribute_enum"}, {"Field Name"="attribute", "Embedded Message Name"="nidaqmx_grpc_ChannelStringAttribute", "Protobuf Index"=3, "MessageElementType"=enum."EnumValue", "Repeated"=FALSE, "Is in Oneof"=TRUE, "Oneof Container Name"="nidaqmx_grpc_GetChanAttributeStringRequest_attribute_enum"}, {"Field Name"="attribute_raw", "Embedded Message Name"="", "Protobuf Index"=4, "MessageElementType"=enum."Int32Value", "Repeated"=FALSE, "Is in Oneof"=TRUE, "Oneof Container Name"="nidaqmx_grpc_GetChanAttributeStringRequest_attribute_enum"}], "Has Oneof"=TRUE}, {"Version"=2, "Name"="nidaqmx_grpc_GetChanAttributeStringResponse", "Type Url"="nidaqmx_grpc.GetChanAttributeStringResponse", "Elements"=[{"Field Name"="status", "Embedded Message Name"="", "Protobuf Index"=1, "MessageElementType"=enum."Int32Value", "Repeated"=FALSE, "Is in Oneof"=FALSE, "Oneof Container Name"=""}, {"Field Name"="value", "Embedded Message Name"="", "Protobuf Index"=2, "MessageElementType"=enum."StringValue", "Repeated"=FALSE, "Is in Oneof"=FALSE, "Oneof Container Name"=""}], "Has Oneof"=FALSE}, {"Version"=2, "Name"="nidaqmx_grpc_GetChanAttributeDoubleRequest", "Type Url"="nidaqmx_grpc.GetChanAttributeDoubleRequest", "Elements"=[{"Field Name"="task", "Embedded Message Name"="nidevice_grpc_Session", "Protobuf Index"=1, "MessageElementType"=enum."MessageValue", "Repeated"=FALSE, "Is in Oneof"=FALSE, "Oneof Container Name"=""}, {"Field Name"="channel", "Embedded Message Name"="", "Protobuf Index"=2, "MessageElementType"=enum."StringValue", "Repeated"=FALSE, "Is in Oneof"=FALSE, "Oneof Container Name"=""}, {"Field Name"="selected_index", "Embedded Message Name"="", "Protobuf Index"=-1, "MessageElementType"=enum."Int32Value", "Repeated"=FALSE, "Is in Oneof"=TRUE, "Oneof Container Name"="nidaqmx_grpc_GetChanAttributeDoubleRequest_attribute_enum"}, {"Field Name"="attribute", "Embedded Message Name"="nidaqmx_grpc_ChannelDoubleAttribute", "Protobuf Index"=3, "MessageElementType"=enum."EnumValue", "Repeated"=FALSE, "Is in Oneof"=TRUE, "Oneof Container Name"="nidaqmx_grpc_GetChanAttributeDoubleRequest_attribute_enum"}, {"Field Name"="attribute_raw", "Embedded Message Name"="", "Protobuf Index"=4, "MessageElementType"=enum."Int32Value", "Repeated"=FALSE, "Is in Oneof"=TRUE, "Oneof Container Name"="nidaqmx_grpc_GetChanAttributeDoubleRequest_attribute_enum"}], "Has Oneof"=TRUE}, {"Version"=2, "Name"="nidaqmx_grpc_GetChanAttributeDoubleResponse", "Type Url"="nidaqmx_grpc.GetChanAttributeDoubleResponse", "Elements"=[{"Field Name"="status", "Embedded Message Name"="", "Protobuf Index"=1, "MessageElementType"=enum."Int32Value", "Repeated"=FALSE, "Is in Oneof"=FALSE, "Oneof Container Name"=""}, {"Field Name"="value", "Embedded Message Name"="", "Protobuf Index"=2, "MessageElementType"=enum."DoubleValue", "Repeated"=FALSE, "Is in Oneof"=FALSE, "Oneof Container Name"=""}], "Has Oneof"=FALSE}, {"Version"=2, "Name"="nidaqmx_grpc_SetChanAttributeStringRequest", "Type Url"="nidaqmx_grpc.SetChanAttributeStringRequest", "Elements"=[{"Field Name"="task", "Embedded Message Name"="nidevice_grpc_Session", "Protobuf Index"=1, "MessageElementType"=enum."MessageValue", "Repeated"=FALSE, "Is in Oneof"=FALSE, "Oneof Container Name"=""}, {"Field Name"="channel", "Embedded Message Name"="", "Protobuf Index"=2, "MessageElementType"=enum."StringValue", "Repeated"=FALSE, "Is in Oneof"=FALSE, "Oneof Container Name"=""}, {"Field Name"="selected_index", "Embedded Message Name"="", "Protobuf Index"=-1, "MessageElementType"=enum."Int32Value", "Repeated"=FALSE, "Is in Oneof"=TRUE, "Oneof Container Name"="nidaqmx_grpc_SetChanAttributeStringRequest_attribute_enum"}, {"Field Name"="attribute", "Embedded Message Name"="nidaqmx_grpc_ChannelStringAttribute", "Protobuf Index"=3, "MessageElementType"=enum."EnumValue", "Repeated"=FALSE, "Is in Oneof"=TRUE, "Oneof Container Name"="nidaqmx_grpc_SetChanAttributeStringRequest_attribute_enum"}, {"Field Name"="attribute_raw", "Embedded Message Name"="", "Protobuf Index"=4, "MessageElementType"=enum."Int32Value", "Repeated"=FALSE, "Is in Oneof"=TRUE, "Oneof Container Name"="nidaqmx_grpc_SetChanAttributeStringRequest_attribute_enum"}, {"Field Name"="value", "Embedded Message Name"="", "Protobuf Index"=5, "MessageElementType"=enum."StringValue", "Repeated"=FALSE, "Is in Oneof"=FALSE, "Oneof Container Name"=""}], "Has Oneof"=TRUE}, {"Version"=2, "Name"="nidaqmx_grpc_SetChanAttributeStringResponse", "Type Url"="nidaqmx_grpc.SetChanAttributeStringResponse", "Elements"=[{"Field Name"="status", "Embedded Message Name"="", "Protobuf Index"=1, "MessageElementType"=enum."Int32Value", "Repeated"=FALSE, "Is in Oneof"=FALSE, "Oneof Container Name"=""}], "Has Oneof"=FALSE}, {"Version"=2, "Name"="nidaqmx_grpc_SetChanAttributeDoubleRequest", "Type Url"="nidaqmx_grpc.SetChanAttributeDoubleRequest", "Elements"=[{"Field Name"="task", "Embedded Message Name"="nidevice_grpc_Session", "Protobuf Index"=1, "MessageElementType"=enum."MessageValue", "Repeated"=FALSE, "Is in Oneof"=FALSE, "Oneof Container Name"=""}, {"Field Name"="channel", "Embedded Message Name"="", "Protobuf Index"=2, "MessageElementType"=enum."StringValue", "Repeated"=FALSE, "Is in Oneof"=FALSE, "Oneof Container Name"=""}, {"Field Name"="selected_index", "Embedded Message Name"="", "Protobuf Index"=-1, "MessageElementType"=enum."Int32Value", "Repeated"=FALSE, "Is in Oneof"=TRUE, "Oneof Container Name"="nidaqmx_grpc_SetChanAttributeDoubleRequest_attribute_enum"}, {"Field Name"="attribute", "Embedded Message Name"="nidaqmx_grpc_ChannelDoubleAttribute", "Protobuf Index"=3, "MessageElementType"=enum."EnumValue", "Repeated"=FALSE, "Is in Oneof"=TRUE, "Oneof Container Name"="nidaqmx_grpc_SetChanAttributeDoubleRequest_attribute_enum"}, {"Field Name"="attribute_raw", "Embedded Message Name"="", "Protobuf Index"=4, "MessageElementType"=enum."Int32Value", "Repeated"=FALSE, "Is in Oneof"=TRUE, "Oneof Container Name"="nidaqmx_grpc_SetChanAttributeDoubleRequest_attribute_enum"}, {"Field Name"="value", "Embedded Message Name"="", "Protobuf Index"=5, "MessageElementType"=enum."DoubleValue", "Repeated"=FALSE, "Is in Oneof"=FALSE, "Oneof Container Name"=""}], "Has Oneof"=TRUE}, {"Version"=2, "Name"="nidaqmx_grpc_SetChanAttributeDoubleResponse", "Type Url"="nidaqmx_grpc.SetChanAttributeDoubleResponse", "Elements"=[{"Field Name"="status", "Embedded Message Name"="", "Protobuf Index"=1, "MessageElementType"=enum."Int32Value", "Repeated"=FALSE, "Is in Oneof"=FALSE, "Oneof Container Name"=""}], "Has Oneof"=FALSE}, {"Version"=2, "Name"="nidevice_grpc_Session", "Type Url"="nidevice_grpc.Session", "Elements"=[{"Field Name"="selected_index", "Embedded Message Name"="", "Protobuf Index"=-1, "MessageElementType"=enum."Int32Value", "Repeated"=FALSE, "Is in Oneof"=TRUE, "Oneof Container Name"="nidevice_grpc_Session_session"}, {"Field Name"="name", "Embedded Message Name"="", "Protobuf Index"=1, "MessageElementType"=enum."StringValue", "Repeated"=FALSE, "Is in Oneof"=TRUE, "Oneof Container Name"="nidevice_grpc_Session_session"}, {"Field Name"="id", "Embedded Message Name"="", "Protobuf Index"=2, "MessageElementType"=enum."UInt32Value", "Repeated"=FALSE, "Is in Oneof"=TRUE, "Oneof Container Name"="nidevice_grpc_Session_session"}], "Has Oneof"=TRUE}, {"Version"=2, "Name"="google_protobuf_Timestamp", "Type Url"="google.protobuf.Timestamp", "Elements"=[{"Field Name"="seconds", "Embedded Message Name"="", "Protobuf Index"=1, "MessageElementType"=enum."Int64Value", "Repeated"=FALSE, "Is in Oneof"=FALSE, "Oneof Container Name"=""}, {"Field Name"="nanos", "Embedded Message Name"="", "Protobuf Index"=2, "MessageElementType"=enum."Int32Value", "Repeated"=FALSE, "Is in Oneof"=FALSE, "Oneof Container Name"=""}], "Has Oneof"=FALSE}]  # Messages MetaData
      n2 = call <vilib>:"Register Message Metadata.vi"("error in"=w10, "Messages"=w11, "gRPCid in"=w9) -> ("error out"=w7:errorcluster, "gRPCid out"=w8:T1)  [unwired: 7 in]
      n3 = call <vilib>:"Register Enum Metadata.vi"("error in"=w7, "Enum Metadata"=w5, "gRPCid in"=w8) -> ("error out"=w6:errorcluster)  [unwired: 7 in, 1 out]
    }
    frame Error {
    }
  }
  "error out" <- w4
  "gRPC ID Out" <- w1
